vi "helper--Button Color Manual.vi"() -> ()   [LabVIEW 2021]
doc: "set the control tags correctly for all of the button types in the directory\n\n<b>Code Developed By:</b>\nTechnology Service Corporation\nwww.tsc.com/atcs\n\nDeveloper:\nDaniel Coons"
panel:
  out "Boolean Text Color read":u32(colorbox)
  out "Colors Array read":cluster{"bg":u32, "fg":u32}[](array[cluster])
  in  "Boolean Text Color":u32(colorbox)
  in  "Colors Array":cluster{"bg":u32, "fg":u32}[](array[cluster])
  in  "write":bool
  in  "Control":u16(ring) items=["elevated--rectangular--icon.ctl", "elevated--rounded--icon.ctl", "filled--rectangular--icon.ctl", "filled--rounded--icon.ctl", "nooutline--rectangular--icon.ctl", "nooutline--rounded--icon.ctl", "outline--rectangular--icon.ctl", "outline--rounded--icon.ctl", "tonal--rectangular--icon.ctl", "tonal--rounded--icon.ctl", "transparent--rectangular--icon.ctl", "transparent--rounded--icon.ctl", "elevated--rectangular--text.ctl", "elevated--rounded--text.ctl", "filled--rectangular--text.ctl", "filled--rounded--text.ctl", "nooutline--rectangular--text.ctl", "nooutline--rounded--text.ctl", "outline--rectangular--text.ctl", "outline--rounded--text.ctl", "tonal--text--rectangular.ctl", "tonal--text--rounded.ctl", "transparent--rectangular--text.ctl", "transparent--rounded--text.ctl", "elevated--rectangular--icon--large.ctl", "elevated--rounded--icon--large.ctl", "filled--rectangular--icon--large.ctl", "filled--rounded--icon--large.ctl", "nooutline--rectangular--icon--large.ctl", "nooutline--rounded--icon--large.ctl", "outline--rectangular--icon--large.ctl", "outline--rounded--icon--large.ctl", "tonal--rectangular--icon--large.ctl", "tonal--rounded--icon--large.ctl", "transparent--rectangular--icon--large.ctl", "transparent--rounded--icon--large.ctl", "elevated--rectangular--text--large.ctl", "elevated--rounded--text--large.ctl", "filled--rectangular--text--large.ctl", "filled--rounded--text--large.ctl", "nooutline--rectangular--text--large.ctl", "nooutline--rounded--text--large.ctl", "outline--rectangular--text--large.ctl", "outline--rounded--text--large.ctl", "tonal--text--rectangular--large.ctl", "tonal--text--rounded--large.ctl", "transparent--rectangular--text--large.ctl", "transparent--rounded--text--large.ctl", "elevated--rectangular--icon--mulitple.ctl", "elevated--rounded--icon--mulitple.ctl", "filled--rectangular--icon--mulitple.ctl", "filled--rounded--icon--mulitple.ctl", "nooutline--rectangular--icon--mulitple.ctl", "nooutline--rounded--icon--mulitple.ctl", "outline--rectangular--icon--mulitple.ctl", "outline--rounded--icon--mulitple.ctl", "tonal--rectangular--icon--mulitple.ctl", "tonal--rounded--icon--mulitple.ctl", "transparent--rectangular--icon--mulitple.ctl", "transparent--rounded--icon--mulitple.ctl", "elevated--rectangular--icon--mulitple--large.ctl", "elevated--rounded--icon--mulitple--large.ctl", "filled--rectangular--icon--mulitple--large.ctl", "filled--rounded--icon--mulitple--large.ctl", "nooutline--rectangular--icon--mulitple--large.ctl", "nooutline--rounded--icon--mulitple--large.ctl", "outline--rectangular--icon--mulitple--large.ctl", "outline--rounded--icon--mulitple--large.ctl", "tonal--rectangular--icon--mulitple--large.ctl", "tonal--rounded--icon--mulitple--large.ctl", "transparent--rectangular--icon--mulitple--large.ctl", "transparent--rounded--icon--mulitple--large.ctl", "FAB--rounded--icon--large.ctl", "FAB--rounded--icon--medium.ctl", "FAB--rounded--icon.ctl", "icon--button--dark.ctl", "icon--button--light.ctl"]
  out "error out":errorcluster
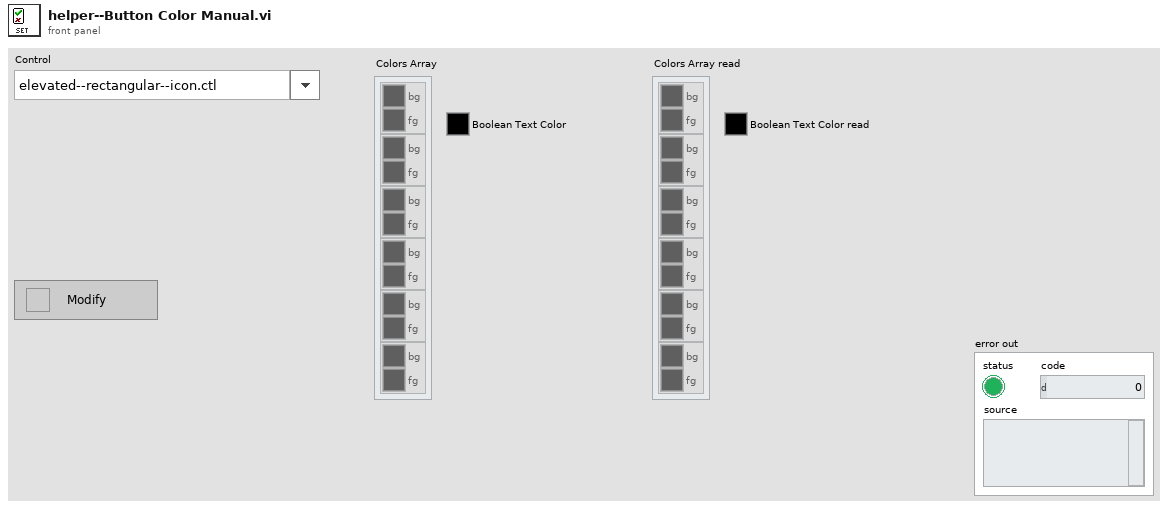
[diagram p1: front panel]
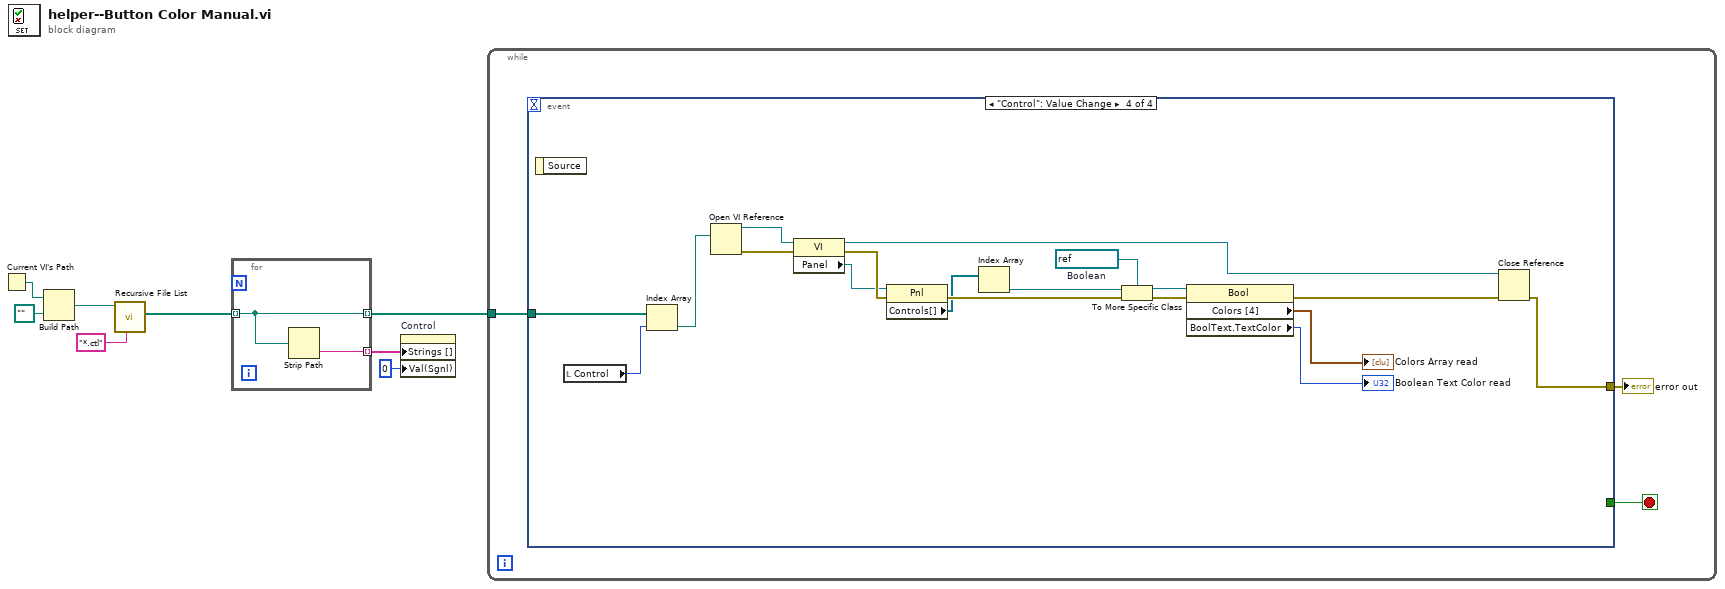
[diagram p0: block diagram]
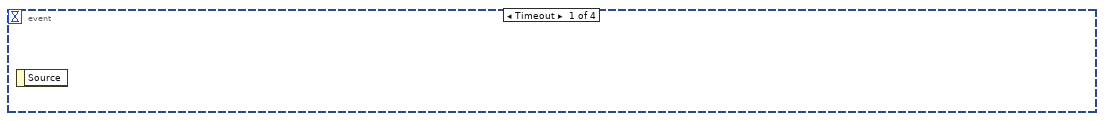
[diagram p2: hidden frame]
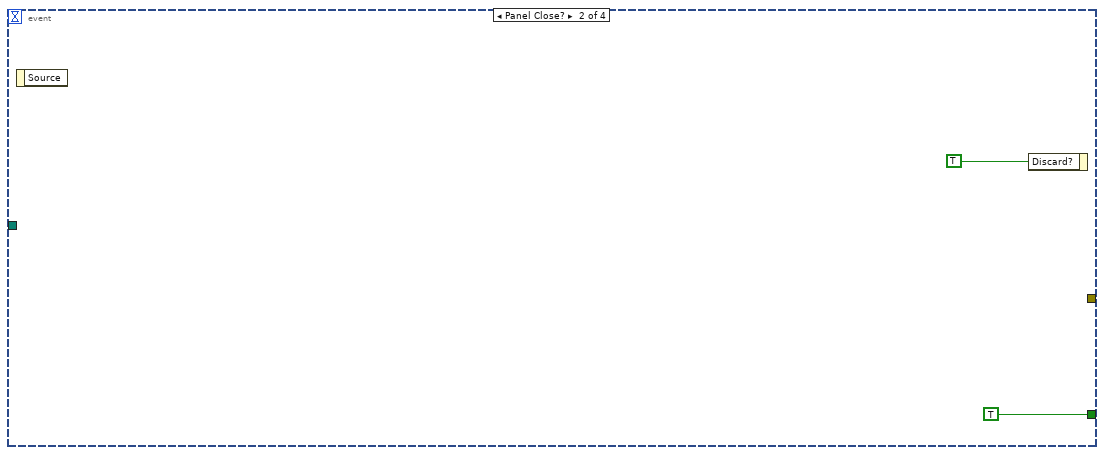
[diagram p3: hidden frame]
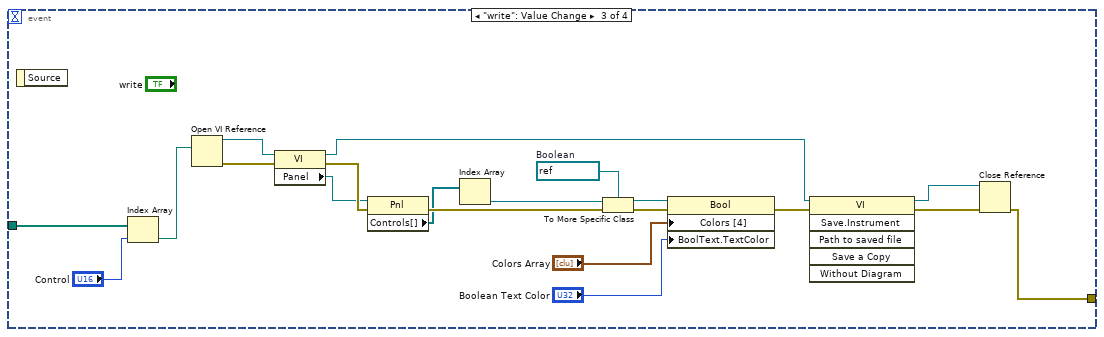
[diagram p4: hidden frame]
diagram:
  n1 = Current VI's Path() -> (path=w8:path)
  n2 = Build Path(base path=w8, name or relative path=path "..") -> (appended path=w6:path)
  n3 = call <vilib>:"Recursive File List.vi"("pattern"="*.ctl", "Folder Path"=w6) -> ("All Files in Dir"=w4:path[])  [unwired: 5 in, 4 out]
  n4 = for {
    tunnel: w4 -> [w10] mode=indexing
    tunnel: [w10] -> w3 mode=indexing
    tunnel: [w9] -> w2 mode=indexing
    n5 = Strip Path(path=w10) -> (name=w9:string)  [unwired: 1 out]
  }
  n6 = property on="Control" class="Ring (strict)"("Strings []"=w2, "Val(Sgnl)"=u16 0 ("Value (Signaling)")) -> ()  [unwired: 2 in, 2 out]
  n7 = while {
    tunnel: w3 -> [w13]
    stop <- w12 stop-if-true
    n8 = event shown="[3] \"Control\": Value Change" {
      selector: _ -> [_ _ _ _]
      dyn-events: _ -> [_ _ _ _]
      timeout: _ -> [_ _ _ _]
      tunnel: [_ _ w24 w44] -> w11
      tunnel: w13 -> [_ _ w25 w45]
      tunnel: [_ TRUE _ _] -> w12
      event Timeout {
        n9 = event-data() -> ()  [unwired: 1 in, 1 out]
      }
      event Panel Close? {
        n10 = event-data() -> ()  [unwired: 1 in, 1 out]
        n11 = event-data("Discard?"=TRUE) -> ()  [unwired: 1 in, 1 out]
      }
      event "write": Value Change {
        w20 = refnum<vi> refnum  # Boolean
        n12 = event-data() -> ()  [unwired: 1 in, 1 out]
        n13 = Index Array(array=w25, index="Control") -> (element=w26:path)
        n14 = Open VI Reference(vi path=w26) -> (vi reference=w33:refnum<vi>, error out=w35:errorcluster)  [unwired: 5 in]
        n15 = property class="VI"(reference=w33, error in=w35) -> (reference out=w28:refnum<vi>, error out=w34:errorcluster, "Panel"=w31:refnum<vi>)
        n16 = property class="Pnl"(reference=w31, error in=w34) -> (error out=w32:errorcluster, "Controls[]"=w30:refnum<vi>[])  [unwired: 1 out]
        n17 = Index Array(array=w30) -> (element=w21:refnum<vi>)  [unwired: 1 in]
        n18 = To More Specific Class(target class=w20, reference=w21, error in=w32) -> (specific class reference=w18:refnum<vi>, error out=w22:errorcluster)
        n19 = property class="Bool"(reference=w18, error in=w22, "Colors [4]"="Colors Array", "BoolText.TextColor"="Boolean Text Color") -> (error out=w19:errorcluster)  [unwired: 1 out]
        n20 = invoke class="VI" method="Save.Instrument"(reference=w28, error in=w19) -> (reference out=w27:refnum<vi>, error out=w29:errorcluster)  [unwired: 4 in, 4 out]
        n21 = Close Reference(reference=w27, error in (no error)=w29) -> (error out=w24:errorcluster)
      }
      event "Control": Value Change {
        w41 = refnum<vi> refnum  # Boolean
        n22 = event-data() -> ()  [unwired: 1 in, 1 out]
        n23 = local read "Control"() -> (w38:u16)
        n24 = Index Array(array=w45, index=w38) -> (element=w46:path)
        n25 = Open VI Reference(vi path=w46) -> (vi reference=w51:refnum<vi>, error out=w53:errorcluster)  [unwired: 5 in]
        n26 = property class="VI"(reference=w51, error in=w53) -> (reference out=w47:refnum<vi>, error out=w52:errorcluster, "Panel"=w49:refnum<vi>)
        n27 = property class="Pnl"(reference=w49, error in=w52) -> (error out=w50:errorcluster, "Controls[]"=w48:refnum<vi>[])  [unwired: 1 out]
        n28 = Index Array(array=w48) -> (element=w42:refnum<vi>)  [unwired: 1 in]
        n29 = To More Specific Class(target class=w41, reference=w42, error in=w50) -> (specific class reference=w39:refnum<vi>, error out=w43:errorcluster)
        n30 = property class="Bool"(reference=w39, error in=w43) -> (error out=w40:errorcluster, "Colors [4]"=→"Colors Array read":cluster{u32, u32}[], "BoolText.TextColor"=→"Boolean Text Color read":u32)  [unwired: 1 out]
        n31 = Close Reference(reference=w47, error in (no error)=w40) -> (error out=w44:errorcluster)
      }
    }
    "error out" <- w11
  }
